vi "parse_speed_is.vi"(8 "error in":errorcluster, 11 "msg in":string) -> (0 "error out":errorcluster, 2 "speed_is":T1, 3 "msg out":string)   [LabVIEW 2016]
uses:
  <userlib>/ROS for LabVIEW Software/ROS/MessageParsing/std_msgs/subs/parse_float64_scalar.vi
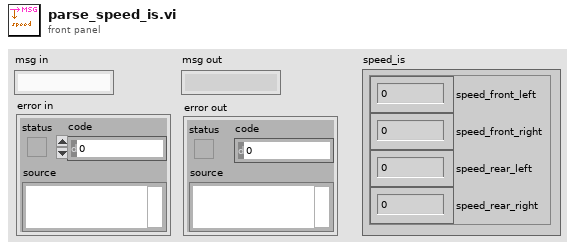
[diagram p1: front panel]
types:
  T1 = cluster{"speed_front_left":dbl, "speed_front_right":dbl, "speed_rear_left":dbl, "speed_rear_right":dbl}
  T2 = cluster{"steering_front_left":dbl, "steering_front_right":dbl, "steering_rear_left":dbl, "steering_rear_right":dbl}
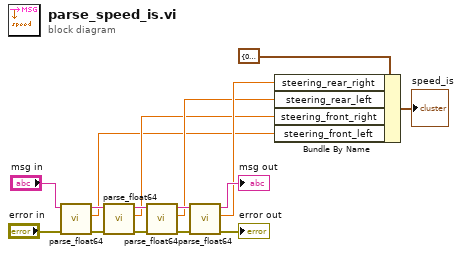
[diagram p0: block diagram]
diagram:
  n1 = call-poly <userlib>:"parse_float64.vi"("error in"="error in", "msg in"="msg in") -> ("error out"=w15:errorcluster, "number"=w3:dbl, "msg out"=w14:string)  [unwired: 3 in]
  n2 = call-poly <userlib>:"parse_float64.vi"("error in"=w15, "msg in"=w14) -> ("error out"=w10:errorcluster, "number"=w4:dbl, "msg out"=w13:string)  [unwired: 3 in]
  n3 = call-poly <userlib>:"parse_float64.vi"("error in"=w10, "msg in"=w13) -> ("error out"=w9:errorcluster, "number"=w5:dbl, "msg out"=w12:string)  [unwired: 3 in]
  n4 = call-poly <userlib>:"parse_float64.vi"("error in"=w9, "msg in"=w12) -> ("error out"=→"error out":errorcluster, "number"=w6:dbl, "msg out"=→"msg out":string)  [unwired: 3 in]
  n5 = Bundle By Name(cluster=T2 {"steering_front_left"=0.0, "steering_front_right"=0.0, "steering_rear_left"=0.0, "steering_rear_right"=0.0}, "steering_rear_right"=w6, "steering_rear_left"=w5, "steering_front_right"=w4, "steering_front_left"=w3) -> (→"speed_is":T2)
